vi "Write time digit.vi"(8 "error in (no error)":errorcluster, 10 "Time":dbl, 11 "Abstract Display in":refnum<class "Abstract Display.lvclass">) -> (0 "error out":errorcluster, 3 "Abstract Display out":refnum<class "Abstract Display.lvclass">)   [LabVIEW 2013, in "Display Panel.lvlib" / "Abstract Display.lvclass"]
uses:
  Abstract Display.lvclass
  Abstract Display.lvclass/Abstract Display.ctl
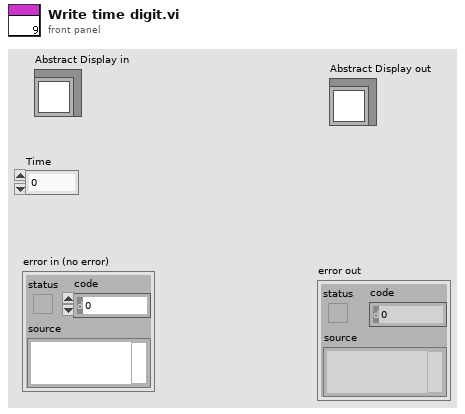
[diagram p1: front panel]
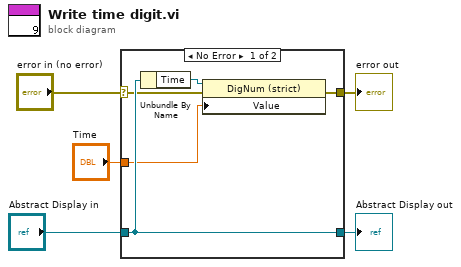
[diagram p0: block diagram]
diagram:
  n1 = case shown="No Error" "error in (no error)" {
    selector: "error in (no error)" -> [w7 w11]
    tunnel: [w6 w11] -> w4
    tunnel: [w10 w12] -> w2
    tunnel: "Abstract Display in" -> [w10 w12]
    tunnel: "Time" -> [w8 _]
    frame No Error {
      n2 = Unbundle By Name(w10) -> ("Time"=w9:refnum<vi>)
      n3 = property class="DigNum (strict)"(reference=w9, error in=w7, "Value"=w8) -> (error out=w6:errorcluster)  [unwired: 1 out]
    }
    frame Error {
    }
  }
  "error out" <- w4
  "Abstract Display out" <- w2
